vi "BRig_dataLC_Selection_PostR_OnOff_l1.vi"() -> (2 "output_Selection_PostR_OnOff":i32)   [LabVIEW 2014]
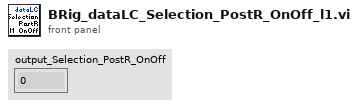
[diagram p1: front panel]
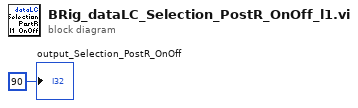
[diagram p0: block diagram]
diagram:
  "output_Selection_PostR_OnOff" <- 90 ("output_iBlock")
